vi "Analysis.Build List of Unique Items, Funct Global, Str.vi"(10 "Item In":string, 11 "Reset":bool) -> (2 "Added":bool, 3 "List Out":string[](array[string]))   [LabVIEW 2024]
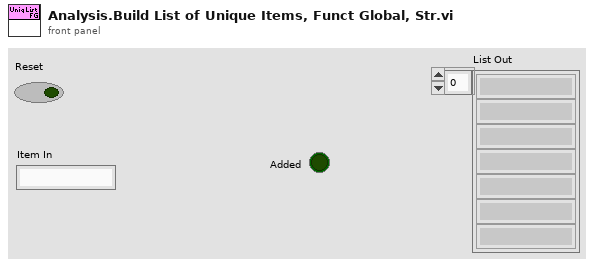
[diagram p1: front panel]
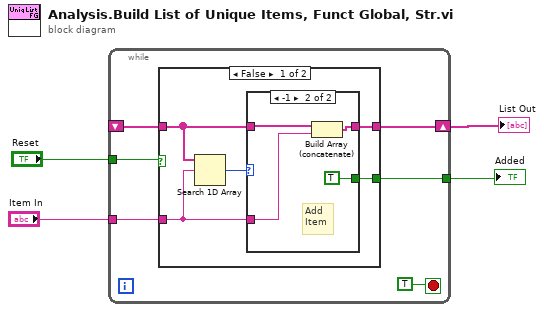
[diagram p0: block diagram]
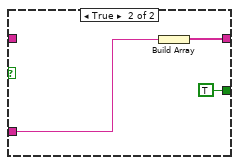
[diagram p3: hidden frame]
diagram:
  n1 = while {
    tunnel: "Item In" -> [w10]
    tunnel: [w7] -> w2
    shift-right: [w9] -> w3
    shift-left: _ -> [w8]
    tunnel: "Reset" -> [w5]
    stop <- TRUE stop-if-true
    n2 = case shown="False" w5 {
      tunnel: w10 -> [w15 w22]
      tunnel: [w14 w23] -> w9
      tunnel: w8 -> [w13 _]
      tunnel: [w11 TRUE] -> w7
      frame False {
        n3 = Search 1D Array(1D array=w13, element=w15) -> (index of element=w12:i32)  [unwired: 1 in]
        n4 = case shown="-1" w12 {
          tunnel: w15 -> [_ w18]
          tunnel: w13 -> [w16 w20]
          tunnel: [w16 w19] -> w14
          tunnel: [_ TRUE] -> w11
          frame Default {
            # "Skip"
          }
          frame -1 {
            # "Add\nItem"
            n5 = Build Array (concatenate)(w20, w18) -> (w19:string[])
          }
        }
      }
      frame True {
        n6 = Build Array(w22) -> (w23:string[])
      }
    }
  }
  "List Out" <- w3
  "Added" <- w2
